vi "Mouse Up.vi"(7 "Map Model in":refnum<class "Map Model.lvclass">, 8 "error in (no error)":errorcluster, 10 "Position":T1, 11 "Line in":refnum<class "Line.lvclass">) -> (0 "error out":errorcluster, 3 "Line out":refnum<class "Line.lvclass">, 5 "Map Model out":refnum<class "Map Model.lvclass">)   [LabVIEW 2020, in "Map Model.lvlib" / "Line.lvclass"]
uses:
  Line.lvclass
  E:/Project/Labview-Projects/Completed projects/Map Editor/Models/Map Model/Tools/Tool/Tool.lvclass
  E:/Project/Labview-Projects/Completed projects/Map Editor/Models/Map Model/Tools/Undoable Tool/Undoable Tool.lvclass
  <vilib>/Utility/miscctls.llb/LVPoint32TypeDef.ctl
  Map Model/Map Model.lvclass
  Tool/Tool.lvclass/Tool.ctl
  Map Model/Map Model.lvclass/Map Model.ctl
  Undoable Tool/Undoable Tool.lvclass/Undoable Tool.ctl
  Undoable Tool/Undoable Tool.lvclass
  Tool/Tool.lvclass
panel:
  # "NOTICE -- YOU MUST LEAVE THIS NOTICE IN PLACE.\n\nCopyright (c) 2017, LIANG LIU Shawn.Liu.cn@gmail.com\nAll rights reserved.\n\nRedistribution and use in source and binary forms, with or without modification, are permitted provided that the following conditions are met:\n-Redistributions of source code must retain the above copyright notice, this list of conditions and the following disclaimer.\n-Redistributions in binary form must reproduce the above copyright notice, this list of conditions and the following disclaimer in the documentation and/or other materials provided with the distribution.\n-Neither the name of the eLp nor the names of its contributors may be used to endorse or promote products derived from this software without specific prior written permission.\n\nTHIS SOFTWARE IS PROVIDED BY THE COPYRIGHT HOLDERS AND CONTRIBUTORS \"AS IS\" AND ANY EXPRESS OR IMPLIED WARRANTIES, INCLUDING, BUT NOT LIMITED TO, THE IMPLIED WARRANTIES OF MERCHANTABILITY AND FITNESS FOR A PARTICULAR PURPOSE ARE DISCLAIMED. IN NO EVENT SHALL THE COPYRIGHT HOLDER OR CONTRIBUTORS BE LIABLE FOR ANY DIRECT, INDIRECT, INCIDENTAL, SPECIAL, EXEMPLARY, OR CONSEQUENTIAL DAMAGES (INCLUDING, BUT NOT LIMITED TO, PROCUREMENT OF SUBSTITUTE GOODS OR SERVICES; LOSS OF USE, DATA, OR PROFITS; OR BUSINESS INTERRUPTION) HOWEVER CAUSED AND ON ANY THEORY OF LIABILITY, WHETHER IN CONTRACT, STRICT LIABILITY, OR TORT (INCLUDING NEGLIGENCE OR OTHERWISE) ARISING IN ANY WAY OUT OF THE USE OF THIS SOFTWARE, EVEN IF ADVISED OF THE POSSIBILITY OF SUCH DAMAGE."
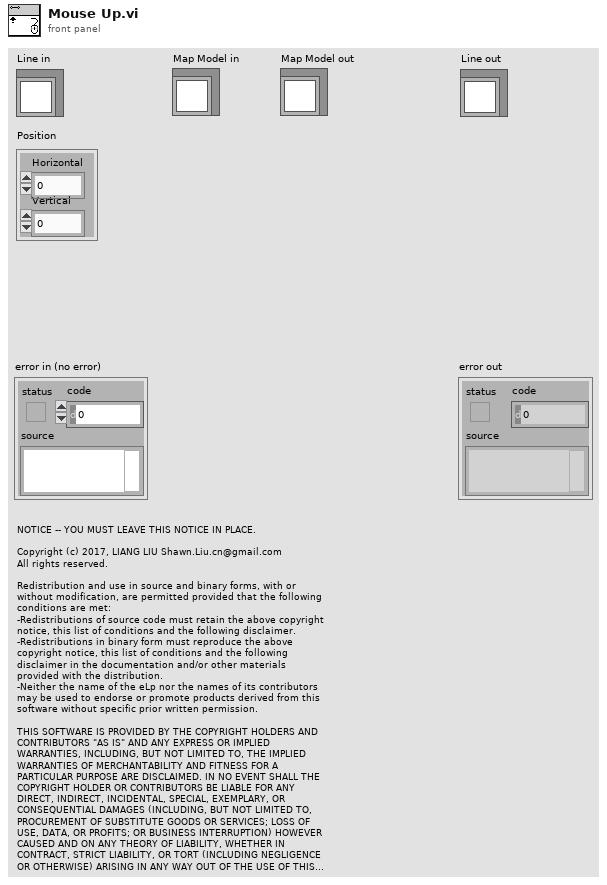
[diagram p1: front panel]
types:
  T1 = typedef "LVPoint32TypeDef.ctl" = cluster{"Horizontal":i32, "Vertical":i32}
  T2 = cluster{"Width":u16, "Style":enum32{"Solid", "Dash", "Dot", "DashDot", "DashDotDot"}}
  T3 = cluster{"Occupied Color":cluster{"Value":u8, "Color":u32}, "Free Color":cluster{"Value":u8, "Color":u32}, "Unknown Color":cluster{"Value":u8, "Color":u32}}
  T4 = typedef "LVPointTypeDef.ctl" = cluster{"Horizontal":i16, "Vertical":i16}
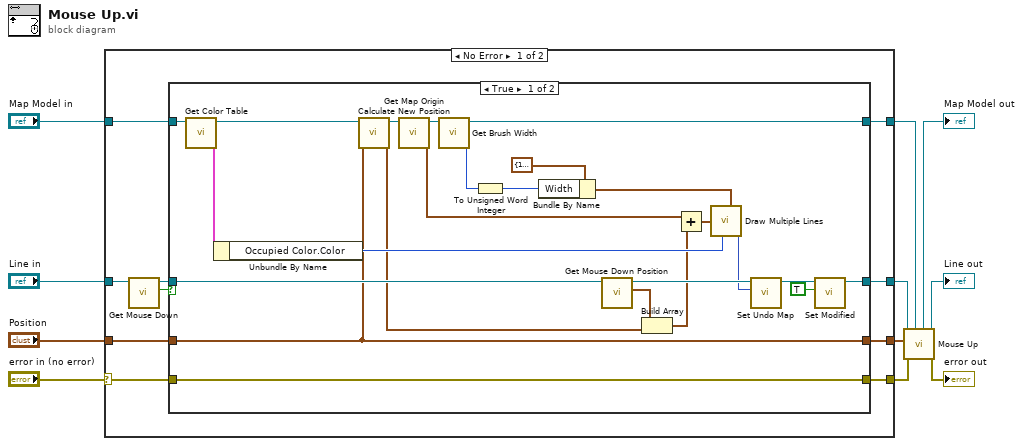
[diagram p0: block diagram]
diagram:
  n1 = case shown="No Error" "error in (no error)" {
    selector: "error in (no error)" -> [w18 w53]
    tunnel: "Map Model in" -> [w21 w52]
    tunnel: "Line in" -> [w20 w51]
    tunnel: "Position" -> [w19 w50]
    tunnel: [w17 w50] -> w7
    tunnel: [w16 w52] -> w6
    tunnel: [w15 w51] -> w5
    tunnel: [w14 w53] -> w2
    frame No Error {
      n2 = call "Get Mouse Down.vi"("Tool in"=w20) -> ("Mouse Down"=w12:bool, "Tool out"=w13:refnum<class "Line.lvclass">)  [unwired: 9 in]
      n3 = case shown="True" w12 {
        tunnel: w13 -> [w45 w49]
        tunnel: w21 -> [w44 w47]
        tunnel: [w42 w47] -> w16
        tunnel: [w23 w49] -> w15
        tunnel: w19 -> [w24 w46]
        tunnel: [w24 w46] -> w17
        tunnel: w18 -> [w32 w48]
        tunnel: [w32 w48] -> w14
        frame True {
          n4 = call "Get Color Table.vi"("Map Model in"=w44) -> ("Color Table"=w38:T3, "Map Model out"=w39:refnum<class "Map Model.lvclass">)  [unwired: 9 in]
          n5 = Unbundle By Name(w38) -> ("Occupied Color.Color"=w36:u32)
          n6 = call "Calculate New Position.vi"("Position in"=w24, "Map Model in"=w39) -> ("Position out"=w25:T1, "Map Model out"=w26:refnum<class "Map Model.lvclass">)  [unwired: 8 in]
          n7 = call "Get Map Origin.vi"("Map Model in"=w26) -> ("Map Origin"=w27:T4, "Map Model out"=w29:refnum<class "Map Model.lvclass">)  [unwired: 9 in]
          n8 = call "Get Brush Width.vi"("Map Model in"=w29) -> ("Brush Width"=w35:i32, "Map Model out"=w42:refnum<class "Map Model.lvclass">)  [unwired: 9 in]
          n9 = To Unsigned Word Integer(number=w35) -> (unsigned 16bit integer=w33:u16)
          n10 = Bundle By Name(cluster=T2 {"Width"=1, "Style"=enum."Solid"} ("pen"), "Width"=w33) -> (w40:T2)
          n11 = call "Get Mouse Down Position.vi"("Tool in"=w45) -> ("Mouse Down Position"=w37:T1, "Tool out"=w43:refnum<class "Line.lvclass">)  [unwired: 9 in]
          n12 = Build Array(w37, w25) -> (w34:T1[])
          n13 = Add(x=w27, y=w34) -> (x+y=w28:T1[])
          n14 = call <vilib>:"Draw Multiple Lines.vi"("line endpoints"=w28, "color(black)"=w36, "pen"=w40) -> ("new picture"=w30:picture)  [unwired: 6 in]
          n15 = call "Set Undo Map.vi"("Undo Map"=w30, "Undoable Tool in"=w43) -> ("Undoable Tool out"=w31:refnum<class "Line.lvclass">)  [unwired: 9 in]
          n16 = call "Set Modified.vi"("Modified"=TRUE, "Tool in"=w31) -> ("Tool out"=w23:refnum<class "Line.lvclass">)  [unwired: 9 in]
        }
        frame False {
        }
      }
    }
    frame Error {
    }
  }
  n17 = call-parent "Mouse Up.vi"("Map Model in"=w6, "error in (no error)"=w2, "Position"=w7, "Undoable Tool in"=w5) -> ("error out"=→"error out":errorcluster, "Undoable Tool out"=→"Line out":refnum<class "Line.lvclass">, "Map Model out"=→"Map Model out":refnum<class "Map Model.lvclass">)  [unwired: 5 in]
